vi "setBentStyle.vi"(0 "reference":refnum<class "ClassRelationshipEdge.lvclass">, 1 "newBentStyle":refnum<class "BentStyle.lvclass">, 5 "error in (no error)":errorcluster) -> (14 "reference out":refnum<class "ClassRelationshipEdge.lvclass">, 19 "error out":errorcluster)   [LabVIEW 2020, in "ClassRelationshipEdge.lvclass"]
doc: "setBentStyle"
uses:
  <resource>/Framework/Providers/Open_GDS/UML/ClassRelationshipEdge_class/ClassRelationshipEdge.lvclass
  <resource>/Framework/Providers/Open_GDS/UML/BentStyle_class/BentStyle.lvclass
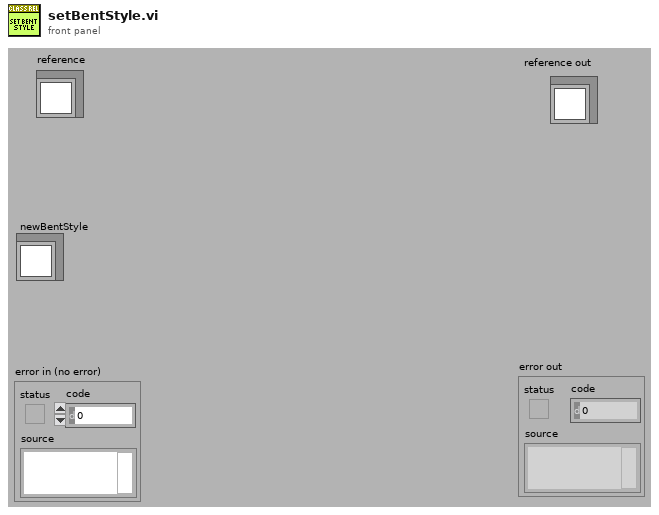
[diagram p1: front panel]
types:
  T1 = typedef "ClassRelationshipEdge.lvclass/ObjectAttributes.ctl" = cluster{"bentStyleRef":refnum<class "BentStyle.lvclass">, "startConnectionOffset":cluster{"x":i32, "y":i32}, "endConnectionOffset":cluster{"x":i32, "y":i32}, "MidLineOffset":cluster{"x":i32, "y":i32}, "DepClass":T2}
  T2 = typedef "ReversedEngineering_ViDependencyDetailsType.ctl" = cluster{"ThisVIs/Ctls":path[], "Dependent_VIs/Ctls":path[]}
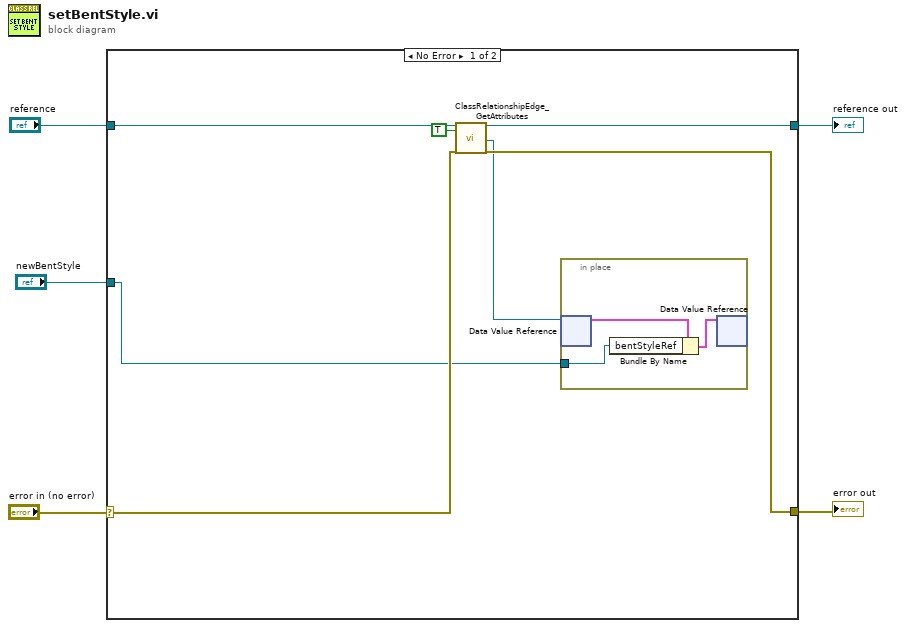
[diagram p0: block diagram]
diagram:
  n1 = case shown="No Error" "error in (no error)" {
    selector: "error in (no error)" -> [w9 w16]
    tunnel: "reference" -> [w12 w17]
    tunnel: [w11 w16] -> w4
    tunnel: [w10 w17] -> w3
    tunnel: "newBentStyle" -> [w6 _]
    frame No Error {
      n2 = call <resource>:"ClassRelationshipEdge_GetAttributes.vi"("reference in"=w12, "OnlyGetDvrReference(False)"=TRUE, "error in (no error)"=w9) -> ("reference out"=w10:refnum<class "ClassRelationshipEdge.lvclass">, "DataRef"=w7:refnum<data-value>, "error out"=w11:errorcluster)  [unwired: 13 in, 1 out]
      n3 = in-place {
        in-place-border: w6 -> [w14]
        n4 = in-place-dvr #1(w7) -> (w15:T1)  [unwired: 1 out]
        n5 = Bundle By Name(cluster=w15, "bentStyleRef"=w14) -> (w13:T1)
        n6 = in-place-dvr #1(w13) -> ()  [unwired: 2 out]
      }
    }
    frame Error {
    }
  }
  "reference out" <- w3
  "error out" <- w4
